vi "Lab2_Acc_Mediat.vi"() -> ()   [LabVIEW 2022 SP3]
uses:
  <vilib>/DAQmx/read.llb/DAQmx Read (Analog 2D DBL NChan NSamp).vi
  <vilib>/DAQmx/miscellaneous.llb/DAQmx Fill In Error Info.vi
panel:
  out "Waveform Mediat":cluster{"data":dbl, "y2":dbl}(graph)
  out "Waveform Chart":cluster{"Waveform":dbl, "Waveform":dbl}[](graph)
  in  "stop":bool
  out "error constant":errorcluster
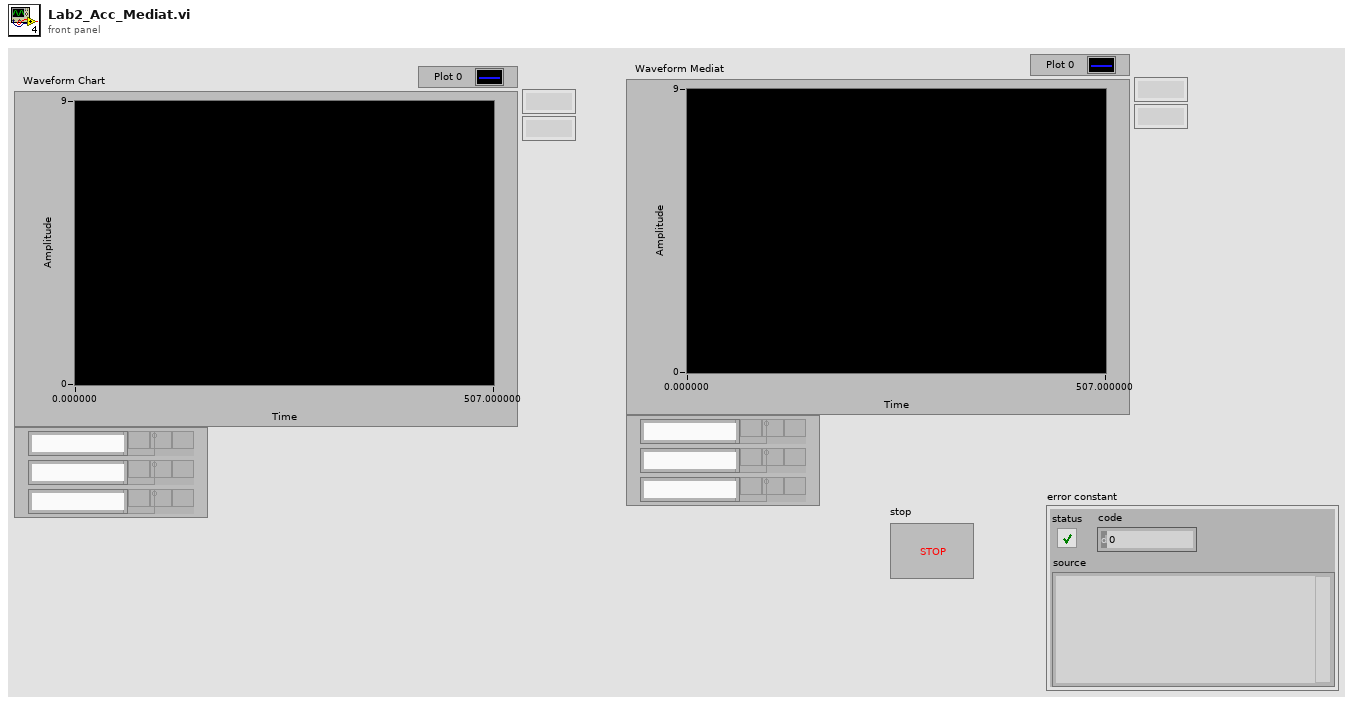
[diagram p1: front panel]
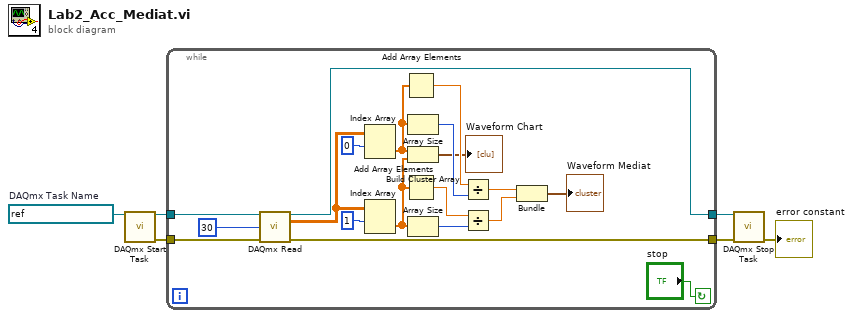
[diagram p0: block diagram]
diagram:
  w2 = refnum<k21> "Accelerometer"  # DAQmx Task Name
  n1 = call <vilib>:"DAQmx Start Task.vi"("task/channels in"=w2) -> ("task out"=w4:refnum<k21>, "error out"=w6:errorcluster)  [unwired: 13 in]
  n2 = while {
    tunnel: w4 -> [w23]
    tunnel: [w22] -> w3
    tunnel: w6 -> [w25]
    tunnel: [w24] -> w5
    stop <- "stop" continue-if-true
    n3 = call-poly <vilib>:"DAQmx Read.vi"("task/channels in"=w23, "number of samples per channel"=30, "error in"=w25) -> ("task out"=w22:refnum<k21>, "data"=w19:dbl[][], "error out"=w24:errorcluster)  [unwired: 10 in]
    n4 = Index Array(array=w19, index (row)=0) -> (element=w8:dbl[])  [unwired: 1 in]
    n5 = Index Array(array=w19, index (row)=1) -> (element=w7:dbl[])  [unwired: 1 in]
    n6 = Add Array Elements(numeric array=w8) -> (sum=w16:dbl)
    n7 = Add Array Elements(numeric array=w7) -> (sum=w13:dbl)
    n8 = Array Size(array=w8) -> (size(s)=w15:i32)
    n9 = Build Cluster Array(w8, w7) -> (→"Waveform Chart":cluster{"Waveform":dbl, "Waveform":dbl}[])
    n10 = Array Size(array=w7) -> (size(s)=w12:i32)
    n11 = Divide(x=w16, y=w15) -> (x/y=w14:dbl)
    n12 = Divide(x=w13, y=w12) -> (x/y=w11:dbl)
    n13 = Bundle(w14, w11) -> (→"Waveform Mediat":cluster{dbl, dbl})  [unwired: 1 in]
  }
  n14 = call <vilib>:"DAQmx Stop Task.vi"("task/channels in"=w3, "error in"=w5) -> ("error out"=→"error constant":errorcluster)  [unwired: 12 in, 1 out]
